vi "ROI grp-Case-Make selected ROIs visible.vi"(8 "error in (no error)":errorcluster) -> (0 "error out":errorcluster)   [LabVIEW 2020]
uses:
  Globals/gl_ROI grp window globals.vi
  <userlib>/_OpenG.lib/array/array.llb/Search 1D Array (String)__ogtk.vi
  <userlib>/_OpenG.lib/array/array.llb/Delete Elements from 1D Array (String)__ogtk.vi
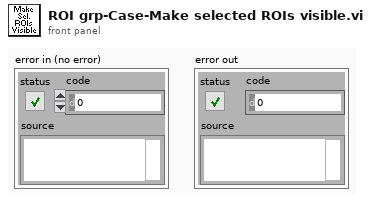
[diagram p1: front panel]
types:
  T1 = typedef "ROI grp-window ctrl refs.ctl" = cluster{"This VI":refnum<vi>, "Pane":refnum<vi>, "Table":refnum<vi>}
  T2 = typedef "LVRowAndColumnTypeDef.ctl" = cluster{"Row":i32, "Column":i32}
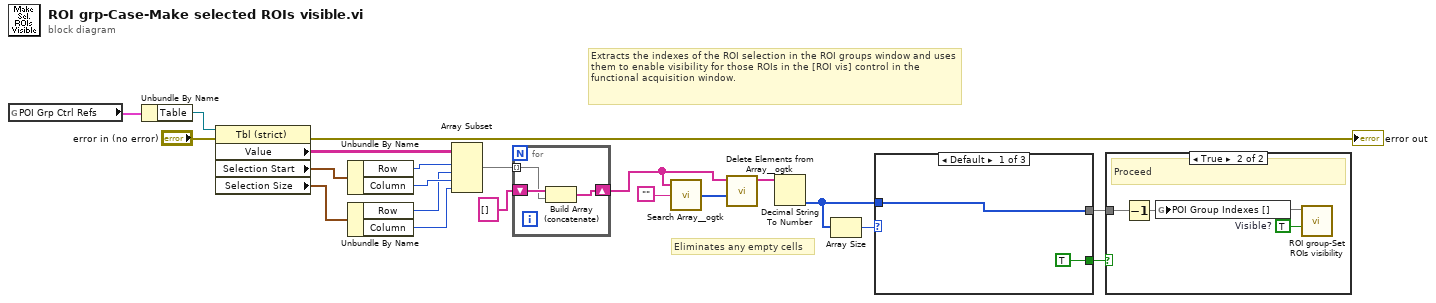
[diagram p0: block diagram]
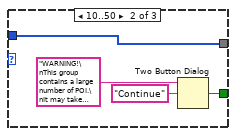
[diagram p3: hidden frame]
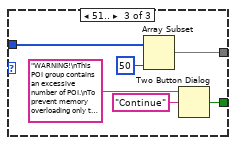
[diagram p4: hidden frame]
diagram:
  # "Extracts the indexes of the ROI selection in the ROI groups window and uses them to enable visibility for those ROIs in the [ROI vis] control in the functional acquisition window."
  # "Eliminates any empty cells"
  n1 = global read "gl_ROI grp window globals.vi" "POI Grp Ctrl Refs"() -> (w3:T1)
  n2 = Unbundle By Name(w3) -> ("Table"=w20:refnum<vi>)
  n3 = property class="Tbl (strict)"(reference=w20, error in="error in (no error)") -> (error out=→"error out":errorcluster, "Value"=w19:string[][], "Selection Start"=w13:T2, "Selection Size"=w10:T2)  [unwired: 1 out]
  n4 = Unbundle By Name(w13) -> ("Row"=w12:i32, "Column"=w11:i32)
  n5 = Unbundle By Name(w10) -> ("Row"=w9:i32, "Column"=w8:i32)
  n6 = Array Subset(array=w19, index (row)=w12, length (row)=w9, index (col)=w11, length (col)=w8) -> (w7:string[][])
  n7 = for {
    tunnel: w7 -> [w23] mode=indexing
    shift-right: [w22] -> w5
    shift-left: string[] [] ("subarray") -> [w24]
    n8 = Build Array (concatenate)(w24, w23) -> (w22:string[])
  }
  n9 = call-poly <userlib>:"Search Array__ogtk.vi"("Array"=w5, "Element Data"="") -> ("Indices of Elements"=w17:i32[])  [unwired: 7 in]
  n10 = call-poly <userlib>:"Delete Elements from Array__ogtk.vi"("indices"=w17, "array"=w5) -> ("array w/ subset deleted"=w16:string[])  [unwired: 8 in, 1 out]
  n11 = Decimal String To Number(string=w16) -> (number=w14:i32[])  [unwired: 2 in, 1 out]
  n12 = Array Size(array=w14) -> (size(s)=w15:i32)
  n13 = case shown="Default" w15 {
    tunnel: [TRUE ("T button?") w28 w35] -> w1
    tunnel: w14 -> [w25 w27 w33]
    tunnel: [w25 w27 w32] -> w4
    frame Default {
    }
    frame 10..50 {
      n14 = Two Button Dialog(message="WARNING!\nThis group contains a large number of POI.\nIt may take some time for the data to be loaded and displayed in the functional imaging viewer screen.", 2:"Continue" ("T button name (\"OK\")")) -> (T button?=w28:bool)  [unwired: 1 in]
    }
    frame 51.. {
      n15 = Array Subset(array=w33, length=50) -> (w32:i32[])  [unwired: 1 in]
      n16 = Two Button Dialog(message="WARNING!\nThis POI group contains an excessive number of POI.\nTo prevent memory overloading only the first 50 POI will be displayed in the graph.\nIt may take some time for the data to be loaded and displayed in the graph.", 2:"Continue" ("T button name (\"OK\")")) -> (T button?=w35:bool)  [unwired: 1 in]
    }
  }
  n17 = case shown="True" w1 {
    tunnel: w4 -> [_ w39]
    frame False {
      # "Cancelled"
    }
    frame True {
      w37 = TRUE  # Visible?
      # "Proceed"
      n18 = Decrement(x=w39) -> (x-1=w38:i32[])
      n19 = global write "gl_ROI grp window globals.vi" "POI Group Indexes []"(w38) -> ()
      n20 = call "ROI group-Set ROIs visibility.vi"("Visible?"=w37, "Indexes of new ROIs to make visible"=w38) -> ()  [unwired: 9 in, 1 out]
    }
  }
